vi "pulse_generator_data_daqmx.vi"(8 "error in":errorcluster) -> (0 "error out":errorcluster, 3 "task out":refnum<k21>)   [LabVIEW 2015]
uses:
  <vilib>/DAQmx/create/channels.llb/DAQmx Create Channel (AI-Voltage-Basic).vi
  <vilib>/DAQmx/create/channels.llb/DAQmx Create Channel (AI-Current-Basic).vi
  <vilib>/DAQmx/create/channels.llb/DAQmx Create Channel (AI-Temperature-Thermocouple).vi
  <resource>/objmgr/daqmx.rc
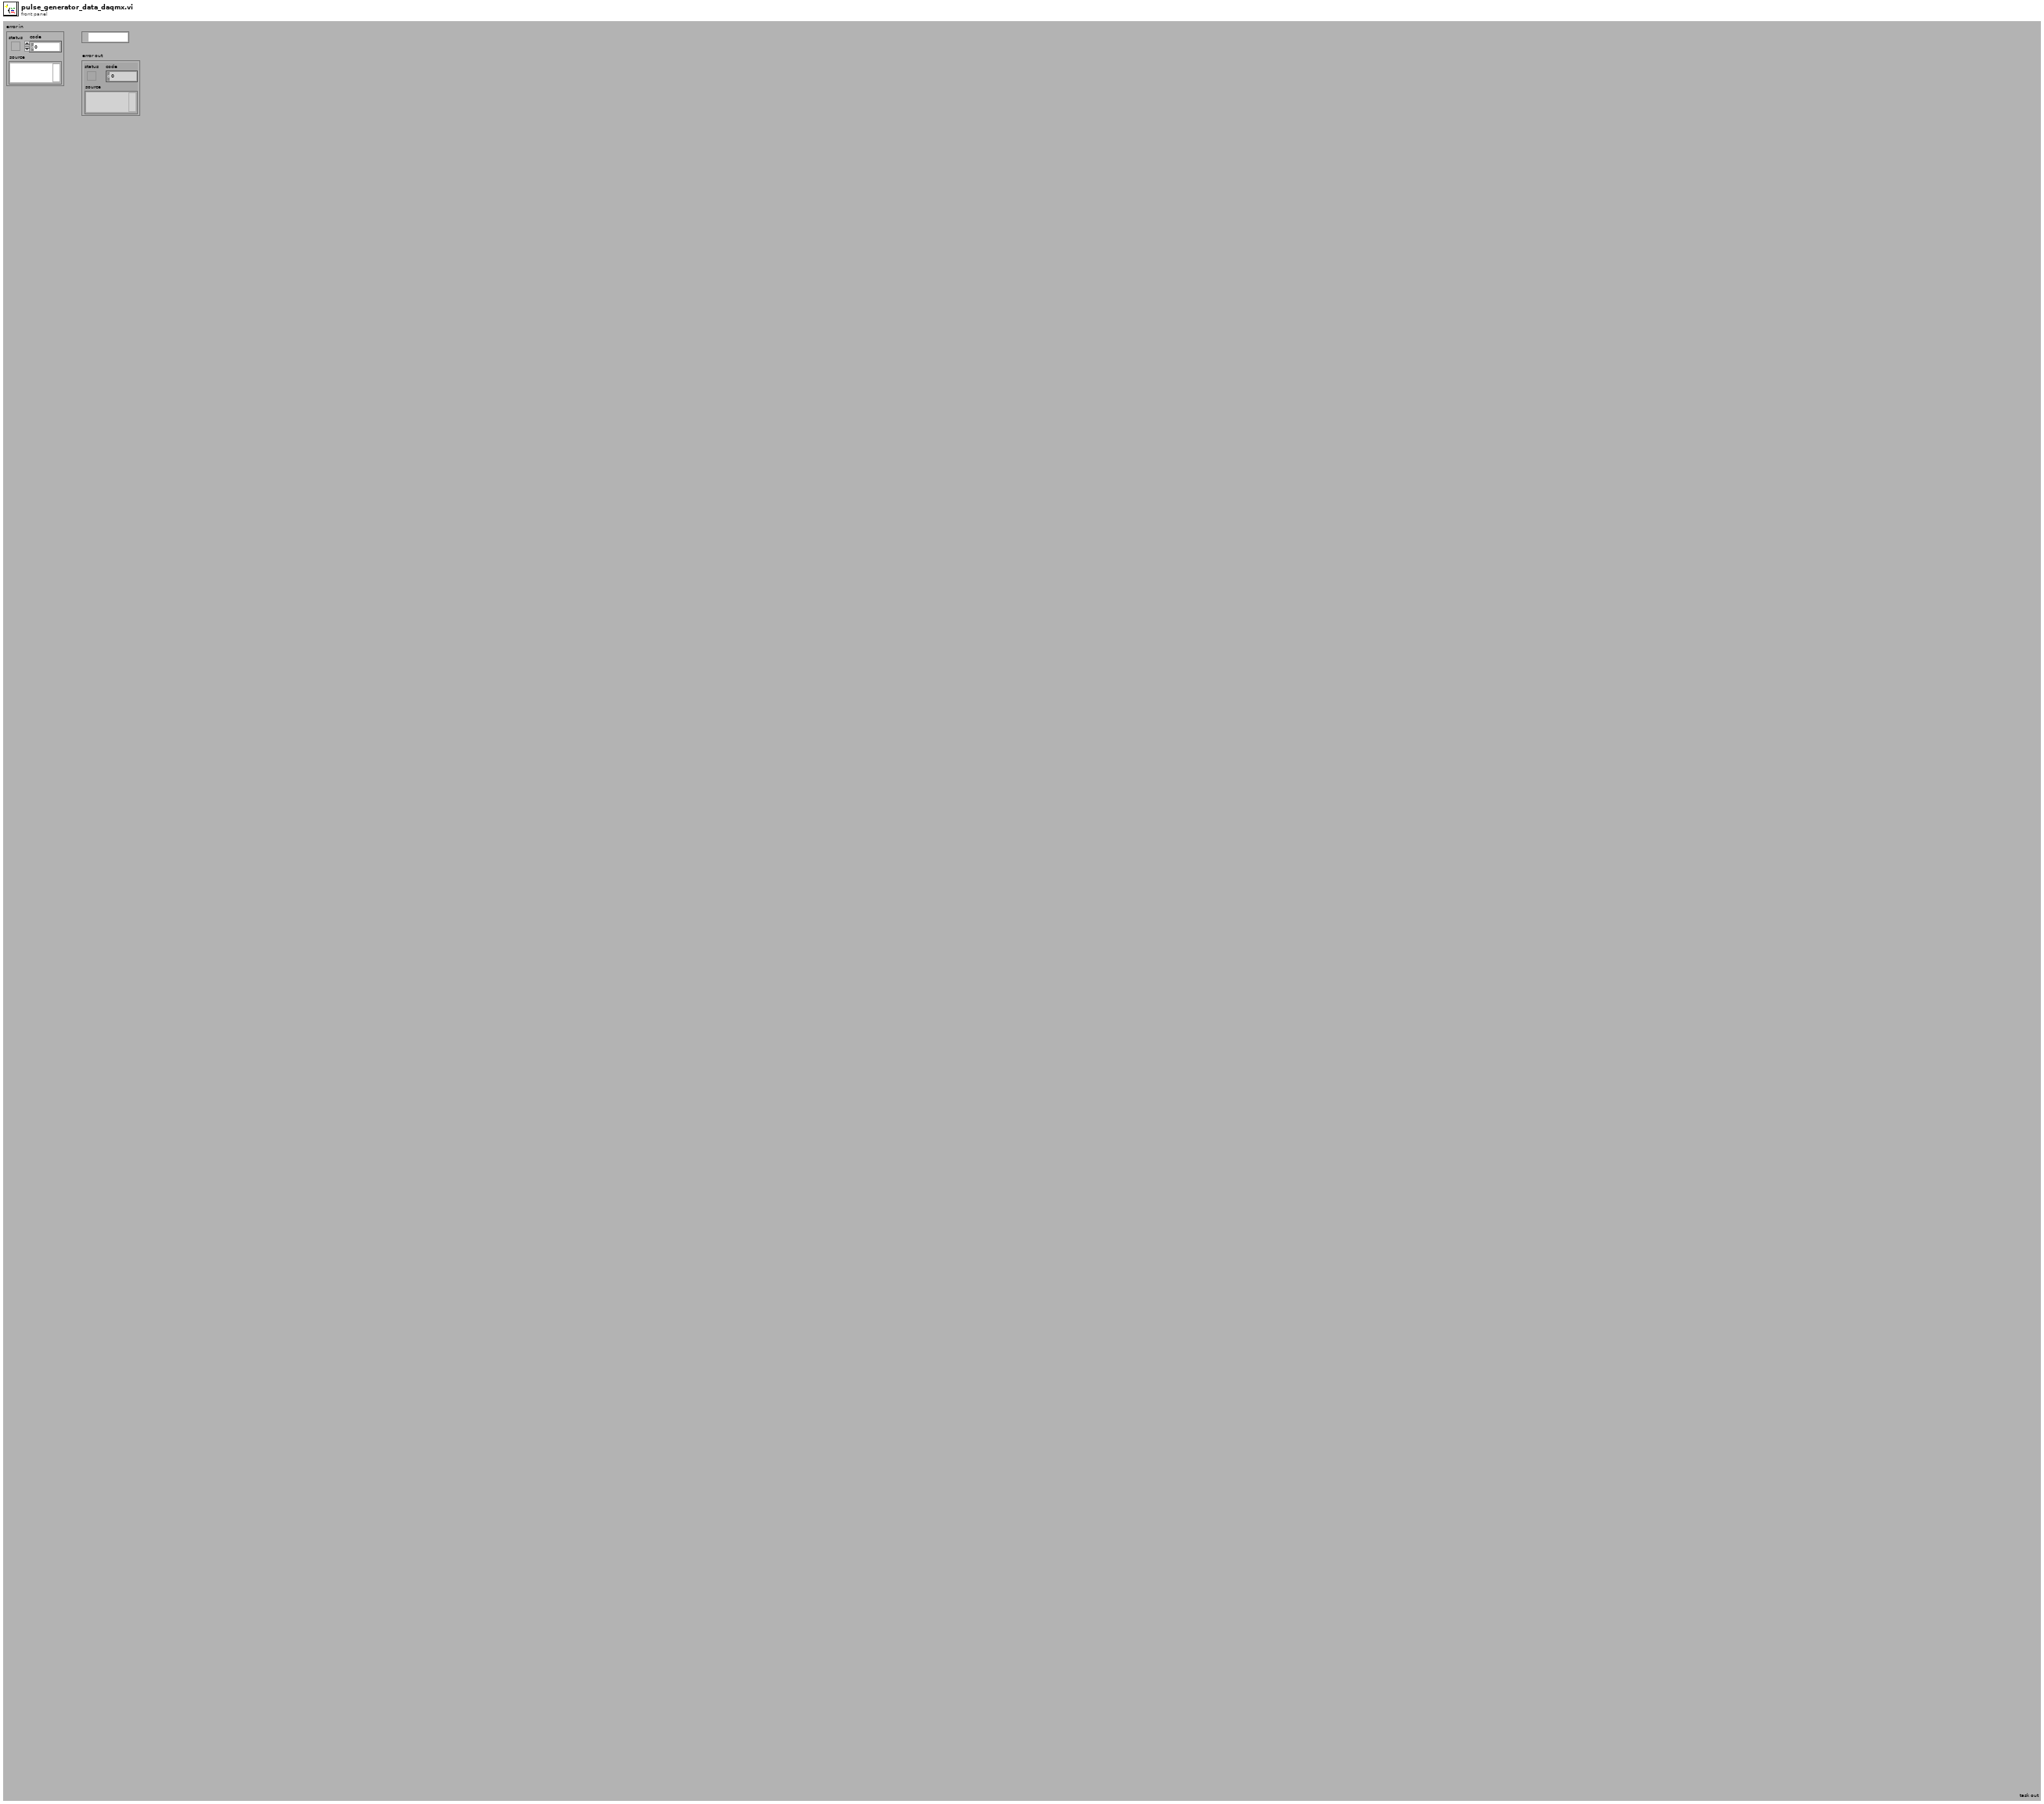
[diagram p1: front panel]
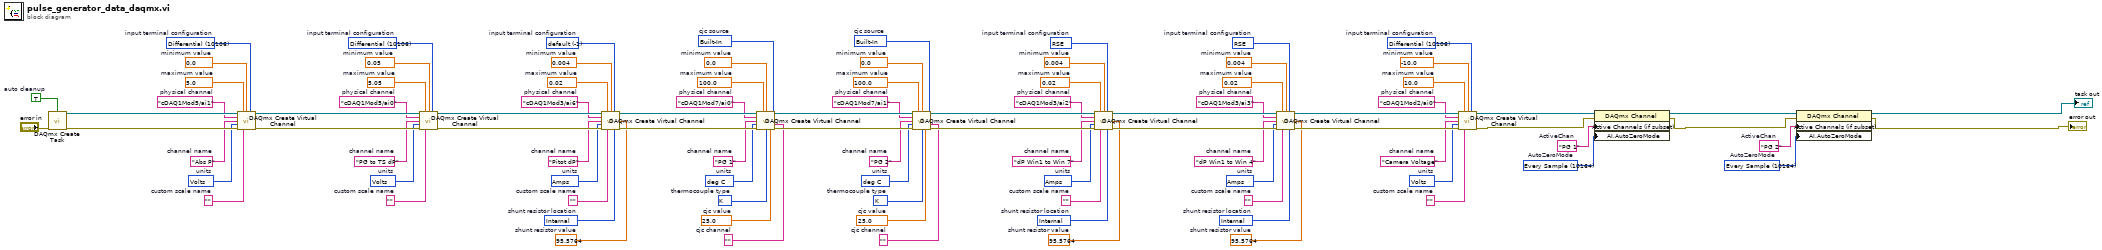
[diagram p0: block diagram]
diagram:
  w3 = 10164 items=["None"=10230, "Once"=10244, "Every Sample"=10164]  # AutoZeroMode
  w5 = "PG 2"  # ActiveChan
  w6 = 10164 items=["None"=10230, "Once"=10244, "Every Sample"=10164]  # AutoZeroMode
  w9 = "PG 1"  # ActiveChan
  w10 = 10106 items=["default"=-1, "RSE"=10083, "NRSE"=10078, "Differential"=10106, "Pseudodifferential"=12529]  # input terminal configuration
  w11 = 10348 items=["Volts"=10348, "From Custom Scale"=10065]  # units
  w12 = "Camera Voltage"  # channel name
  w14 = ""  # custom scale name
  w15 = -10.0  # minimum value
  w16 = 10.0  # maximum value
  w17 = "cDAQ1Mod2/ai0"  # physical channel
  w19 = 10083 items=["default"=-1, "RSE"=10083, "NRSE"=10078, "Differential"=10106, "Pseudodifferential"=12529]  # input terminal configuration
  w20 = 10342 items=["Amps"=10342, "From Custom Scale"=10065]  # units
  w21 = 95.5764  # shunt resistor value
  w22 = 10200 items=["Internal"=10200, "External"=10167]  # shunt resistor location
  w23 = "dP Win1 to Win 4"  # channel name
  w25 = ""  # custom scale name
  w26 = 0.004  # minimum value
  w27 = 0.02  # maximum value
  w28 = "cDAQ1Mod3/ai3"  # physical channel
  w30 = 10083 items=["default"=-1, "RSE"=10083, "NRSE"=10078, "Differential"=10106, "Pseudodifferential"=12529]  # input terminal configuration
  w31 = 10342 items=["Amps"=10342, "From Custom Scale"=10065]  # units
  w32 = 95.5764  # shunt resistor value
  w33 = 10200 items=["Internal"=10200, "External"=10167]  # shunt resistor location
  w34 = "dP Win1 to Win 7"  # channel name
  w36 = ""  # custom scale name
  w37 = 0.004  # minimum value
  w38 = 0.02  # maximum value
  w39 = "cDAQ1Mod3/ai2"  # physical channel
  w41 = 10200 items=["Built-In"=10200, "Constant Value"=10116, "Channel"=10113]  # cjc source
  w43 = ""  # cjc channel
  w44 = 25.0  # cjc value
  w45 = 10073 items=["J"=10072, "K"=10073, "N"=10077, "R"=10082, "S"=10085, "T"=10086, "B"=10047, "E"=10055]  # thermocouple type
  w46 = 10143 items=["deg C"=10143, "deg F"=10144, "Kelvins"=10325, "deg R"=10145, "From Custom Scale"=10065]  # units
  w42 = "PG 2"  # channel name
  w48 = 0.0  # minimum value
  w49 = 100.0  # maximum value
  w50 = "cDAQ1Mod7/ai1"  # physical channel
  w52 = 10200 items=["Built-In"=10200, "Constant Value"=10116, "Channel"=10113]  # cjc source
  w54 = ""  # cjc channel
  w55 = 25.0  # cjc value
  w56 = 10073 items=["J"=10072, "K"=10073, "N"=10077, "R"=10082, "S"=10085, "T"=10086, "B"=10047, "E"=10055]  # thermocouple type
  w57 = 10143 items=["deg C"=10143, "deg F"=10144, "Kelvins"=10325, "deg R"=10145, "From Custom Scale"=10065]  # units
  w53 = "PG 1"  # channel name
  w59 = 0.0  # minimum value
  w60 = 100.0  # maximum value
  w61 = "cDAQ1Mod7/ai0"  # physical channel
  w63 = -1 items=["default"=-1, "RSE"=10083, "NRSE"=10078, "Differential"=10106, "Pseudodifferential"=12529]  # input terminal configuration
  w64 = 10342 items=["Amps"=10342, "From Custom Scale"=10065]  # units
  w65 = 95.5764  # shunt resistor value
  w66 = 10200 items=["Internal"=10200, "External"=10167]  # shunt resistor location
  w67 = "Pitot dP"  # channel name
  w69 = ""  # custom scale name
  w70 = 0.004  # minimum value
  w71 = 0.02  # maximum value
  w72 = "cDAQ1Mod3/ai6"  # physical channel
  w74 = 10106 items=["default"=-1, "RSE"=10083, "NRSE"=10078, "Differential"=10106, "Pseudodifferential"=12529]  # input terminal configuration
  w75 = 10348 items=["Volts"=10348, "From Custom Scale"=10065]  # units
  w76 = "PG to TS dP"  # channel name
  w78 = ""  # custom scale name
  w79 = 0.05  # minimum value
  w80 = 5.05  # maximum value
  w81 = "cDAQ1Mod5/ai0"  # physical channel
  w83 = 10106 items=["default"=-1, "RSE"=10083, "NRSE"=10078, "Differential"=10106, "Pseudodifferential"=12529]  # input terminal configuration
  w84 = 10348 items=["Volts"=10348, "From Custom Scale"=10065]  # units
  w85 = "Abs P"  # channel name
  w87 = ""  # custom scale name
  w88 = 0.0  # minimum value
  w89 = 5.0  # maximum value
  w90 = "cDAQ1Mod5/ai1"  # physical channel
  w92 = TRUE  # auto cleanup
  n1 = call <vilib>:"DAQmx Create Task.vi"("auto cleanup"=w92, "error in"="error in") -> ("task out"=w91:refnum<k21>, "error out"=w93:errorcluster)  [unwired: 12 in]
  n2 = call-poly <vilib>:"DAQmx Create Virtual Channel.vi"("task in"=w91, "maximum value"=w89, "minimum value"=w88, "input terminal configuration"=w83, "physical channels"=w90, "name to assign"=w85, "units"=w84, "error in"=w93, "custom scale name"=w87) -> ("task out"=w82:refnum<k21>, "error out"=w86:errorcluster)  [unwired: 5 in]
  n3 = call-poly <vilib>:"DAQmx Create Virtual Channel.vi"("task in"=w82, "maximum value"=w80, "minimum value"=w79, "input terminal configuration"=w74, "physical channels"=w81, "name to assign"=w76, "units"=w75, "error in"=w86, "custom scale name"=w78) -> ("task out"=w73:refnum<k21>, "error out"=w77:errorcluster)  [unwired: 5 in]
  n4 = call-poly <vilib>:"DAQmx Create Virtual Channel.vi"("task in"=w73, "maximum value"=w71, "minimum value"=w70, "input terminal configuration"=w63, "physical channels"=w72, "name to assign"=w67, "external shunt resistor value"=w65, "units"=w64, "error in"=w77, "custom scale name"=w69, "shunt resistor location"=w66) -> ("task out"=w62:refnum<k21>, "error out"=w68:errorcluster)  [unwired: 3 in]
  n5 = call-poly <vilib>:"DAQmx Create Virtual Channel.vi"("task in"=w62, "maximum value"=w60, "minimum value"=w59, "physical channels"=w61, "cjc source"=w52, "name to assign"=w53, "units"=w57, "cjc channel"=w54, "error in"=w68, "thermocouple type"=w56, "cjc value"=w55) -> ("task out"=w51:refnum<k21>, "error out"=w58:errorcluster)  [unwired: 3 in]
  n6 = call-poly <vilib>:"DAQmx Create Virtual Channel.vi"("task in"=w51, "maximum value"=w49, "minimum value"=w48, "physical channels"=w50, "cjc source"=w41, "name to assign"=w42, "units"=w46, "cjc channel"=w43, "error in"=w58, "thermocouple type"=w45, "cjc value"=w44) -> ("task out"=w40:refnum<k21>, "error out"=w47:errorcluster)  [unwired: 3 in]
  n7 = call-poly <vilib>:"DAQmx Create Virtual Channel.vi"("task in"=w40, "maximum value"=w38, "minimum value"=w37, "input terminal configuration"=w30, "physical channels"=w39, "name to assign"=w34, "external shunt resistor value"=w32, "units"=w31, "error in"=w47, "custom scale name"=w36, "shunt resistor location"=w33) -> ("task out"=w29:refnum<k21>, "error out"=w35:errorcluster)  [unwired: 3 in]
  n8 = call-poly <vilib>:"DAQmx Create Virtual Channel.vi"("task in"=w29, "maximum value"=w27, "minimum value"=w26, "input terminal configuration"=w19, "physical channels"=w28, "name to assign"=w23, "external shunt resistor value"=w21, "units"=w20, "error in"=w35, "custom scale name"=w25, "shunt resistor location"=w22) -> ("task out"=w18:refnum<k21>, "error out"=w24:errorcluster)  [unwired: 3 in]
  n9 = call-poly <vilib>:"DAQmx Create Virtual Channel.vi"("task in"=w18, "maximum value"=w16, "minimum value"=w15, "input terminal configuration"=w10, "physical channels"=w17, "name to assign"=w12, "units"=w11, "error in"=w24, "custom scale name"=w14) -> ("task out"=w7:refnum<k21>, "error out"=w13:errorcluster)  [unwired: 5 in]
  n10 = property class="DAQmx Channel"(reference=w7, error in=w13, "Active Channels (if subset)"=w9, "AI.AutoZeroMode"=w6) -> (reference out=w4:refnum<k21>, error out=w8:errorcluster)
  n11 = property class="DAQmx Channel"(reference=w4, error in=w8, "Active Channels (if subset)"=w5, "AI.AutoZeroMode"=w3) -> (reference out=→"task out":refnum<k21>, error out=→"error out":errorcluster)
